vi "数据输出.vi"(8 "error in (no error)":errorcluster caption="错误输入（无错误）", 11 "SingleStepTestV3 输入":refnum<class "SingleStepCODMnV2.lvclass">) -> (0 "error out":errorcluster caption="错误输出", 2 "data":T1, 3 "SingleStepTestV3 输出":refnum<class "SingleStepCODMnV2.lvclass">)   [LabVIEW 2022 SP3, in "SingleStepCODMnV2.lvlib" / "SingleStepCODMnV2.lvclass"]
uses:
  SingleStepCODMnV2.lvclass
  SingleStepCODMnV2.lvclass/SingleStepCODMnV2.ctl
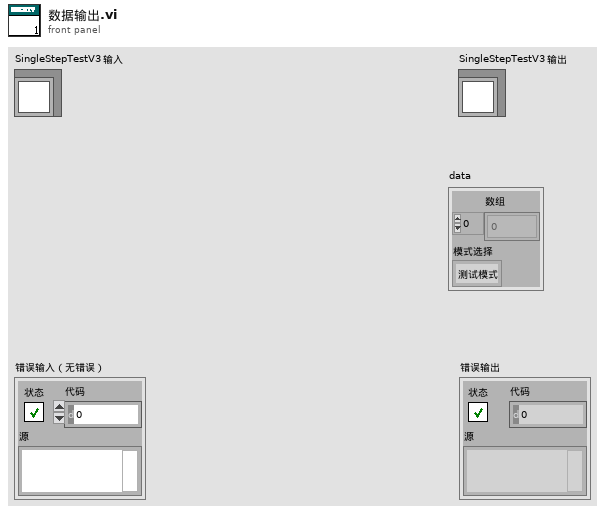
[diagram p1: front panel]
types:
  T1 = cluster{"数组":u16[], "模式选择":enum16{"测试模式", "流程模式"}}
  T2 = typedef "SingleStepCODMnV2.lvlib/SingleStepCODMnV2.lvclass/State Data.ctl" = cluster{"data":u16[], "模式选择":enum16{"测试模式", "流程模式"}}
  T3 = cluster{"data":u16[], "模式选择":enum16{"测试模式", "流程模式"}}
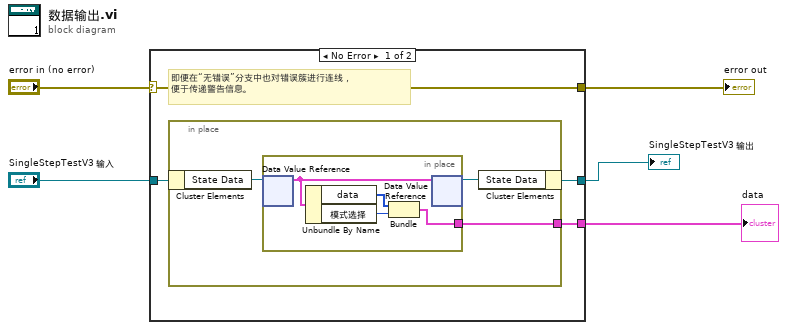
[diagram p0: block diagram]
diagram:
  n1 = case shown="No Error" "error in (no error)" {
    selector: "error in (no error)" -> [w9 w18]
    tunnel: [w9 w18] -> w4
    tunnel: [w7 w17] -> w2
    tunnel: "SingleStepTestV3 输入" -> [w8 w17]
    tunnel: [w6 _] -> w1
    frame No Error {
      # "即便在“无错误”分支中也对错误簇进行连线，\n便于传递警告信息。"
      n2 = in-place {
        in-place-border: [w10] -> w6
        n3 = in-place-cluster #1(w8) -> ("State Data"=w12:refnum<data-value>)
        n4 = in-place {
          in-place-border: [w13] -> w10
          n5 = in-place-dvr #2(w12) -> (w16:T2)  [unwired: 1 out]
          n6 = Unbundle By Name(w16) -> ("data"=w15:u16[], "模式选择"=w14:enum16{"测试模式", "流程模式"})
          n7 = Bundle("data"=w15, "模式选择"=w14) -> (w13:T3)  [unwired: 1 in]
          n8 = in-place-dvr #2(w16) -> (w11:refnum<data-value>)  [unwired: 1 out]
        }
        n9 = in-place-cluster #1("State Data"=w11) -> (w7:refnum<class "SingleStepCODMnV2.lvclass">)
      }
    }
    frame Error {
    }
  }
  "error out" <- w4
  "SingleStepTestV3 输出" <- w2
  "data" <- w1
